vi "Get Step Parameter.vi"(0 "VISA resource name":refnum<visa-resource-name>, 7 "Step Number (0 = Active Step)":i32, 11 "error in (no error)":errorcluster) -> (4 "VISA resource name out":refnum<visa-resource-name>, 8 "Step Parameter":string, 15 "error out":errorcluster)   [LabVIEW 2012, in "Associated Research 78XX Series.lvlib"]
doc: "LS <step number>?\nLists all the parameters for the individual step indicated by step number.\n\nThe response will be formatted as follows; <Step, test, p1, p2, p3.. >\nwhere\n<step> is the step number\n<test> is the test type\n<p1,p2,..> indicates the pareameters of the test"
uses:
  <instrlib>/Associated Research 78XX Series/Associated Research 78XX Series.lvlib
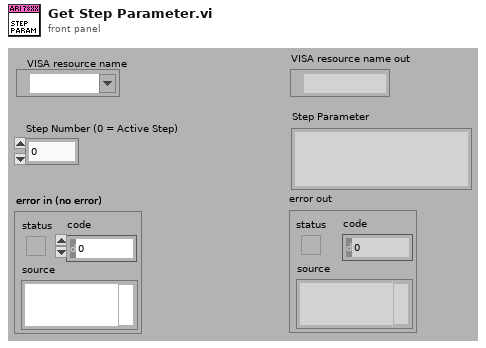
[diagram p1: front panel]
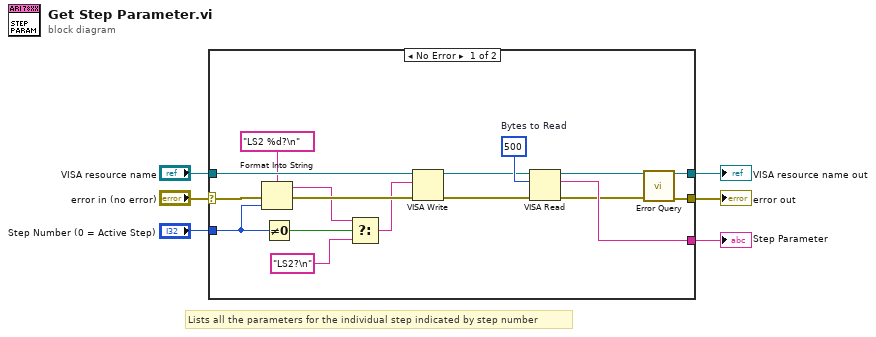
[diagram p0: block diagram]
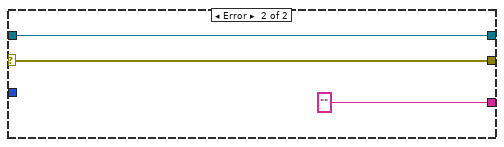
[diagram p2: hidden frame]
diagram:
  # "Lists all the parameters for the individual step indicated by step number"
  n1 = case shown="No Error" "error in (no error)" {
    selector: "error in (no error)" -> [w12 w26]
    tunnel: [w21 w26] -> w5
    tunnel: [w23 w25] -> w3
    tunnel: "VISA resource name" -> [w13 w25]
    tunnel: "Step Number (0 = Active Step)" -> [w19 _]
    tunnel: [w16 "" ("read buffer")] -> w1
    frame No Error {
      w9 = u32 500  # Bytes to Read
      n2 = Format Into String(format string="LS2 %d?\n" ("\"False\" Command"), error in=w12, w19) -> (resulting string=w17:string, error out=w22:errorcluster)  [unwired: 1 in]
      n3 = Not Equal To 0?(x=w19) -> (x != 0?=w20:bool)
      n4 = Select(t=w17, s=w20, f="LS2?\n") -> (s? t:f=w18:string)
      n5 = VISA Write(VISA resource name=w13, write buffer=w18, error in (no error)=w22) -> (VISA resource name out=w7:refnum<visa-resource-name>, error out=w8:errorcluster)  [unwired: 1 out]
      n6 = VISA Read(VISA resource name=w7, byte count=w9, error in (no error)=w8) -> (VISA resource name out=w14:refnum<visa-resource-name>, read buffer=w16:string, error out=w15:errorcluster)  [unwired: 1 out]
      n7 = call <instrlib>:"Error Query.vi"("VISA resource name"=w14, "error in (no error)"=w15) -> ("VISA resource name out"=w23:refnum<visa-resource-name>, "error out"=w21:errorcluster)  [unwired: 10 in, 2 out]
    }
    frame Error {
    }
  }
  "error out" <- w5
  "VISA resource name out" <- w3
  "Step Parameter" <- w1
